vi "basic - Board Configuration.vi"() -> ()   [LabVIEW 2020]
uses:
  _controls/initialize_ExpertMode.ctl
  _controls/initialize_PortSpeed.ctl
  _controls/initialize_PortConfig.ctl
  AIM664LV.lvlib
panel:
  out "BSP Version Parameters":string[][](table)
  in  "ARINC 664 Resources":string[](tree)
  in  "Server Name":string="local"
  out "NuOfResources":u32
  out "new config":bool
  out "Board Control Out":T1 {"SharedMemFree" format="%x"; "GlobalMemFree" format="%x"; "ExpertMode" items=["FDX_EXPERT_MODE", "FDX_DISA_GHOST"]; "PortGoodLink" items=["FDX_NO_LINK", "FDX_GOOD_LINK"]; "PortSpeed" items=["FDX_100MBIT", "FDX_10MBIT", "FDX_AUTO_100MBIT", "FDX_AUTO_10MBIT", "FDX_AUTO_ERROR", "FDX_1000MBIT"]; "PortConfig" items=["FDX_SINGLE", "FDX_REDUNDANT"]}
  out "BSP Version Out":T2
  out "timed out":bool
  in  "PortConfig (single)":T3 {"Port1ConfigIn" items=["FDX_SINGLE", "FDX_REDUNDANT"]; "Port2ConfigIn" items=["FDX_SINGLE", "FDX_REDUNDANT"]; "Port3ConfigIn" items=["FDX_SINGLE", "FDX_REDUNDANT"]; "Port4ConfigIn" items=["FDX_SINGLE", "FDX_REDUNDANT"]}
  in  "PortSpeed (100Mbit)":T4 {"Port4SpeedIn" items=["FDX_100MBIT"=0, "FDX_10MBIT"=1, "FDX_AUTO_100MBIT"=2, "FDX_AUTO_10MBIT"=3, "FDX_1000MBIT"=5]; "Port3SpeedIn" items=["FDX_100MBIT"=0, "FDX_10MBIT"=1, "FDX_AUTO_100MBIT"=2, "FDX_AUTO_10MBIT"=3, "FDX_1000MBIT"=5]; "Port2SpeedIn" items=["FDX_100MBIT"=0, "FDX_10MBIT"=1, "FDX_AUTO_100MBIT"=2, "FDX_AUTO_10MBIT"=3, "FDX_1000MBIT"=5]; "Port1SpeedIn" items=["FDX_100MBIT"=0, "FDX_10MBIT"=1, "FDX_AUTO_100MBIT"=2, "FDX_AUTO_10MBIT"=3, "FDX_1000MBIT"=5]}
  in  "ExpertMode(ExpertMode)":T5 {"Expert1Mode" items=["FDX_EXPERT_MODE", "FDX_DISA_GHOST"]; "Expert2Mode" items=["FDX_EXPERT_MODE", "FDX_DISA_GHOST"]; "Expert3Mode" items=["FDX_EXPERT_MODE", "FDX_DISA_GHOST"]; "Expert4Mode" items=["FDX_EXPERT_MODE", "FDX_DISA_GHOST"]}
  out "error out":errorcluster
  in  "board index":i32
  # "ARINC 664 Board Control"
  # "Overview: Queries the boards available in a system and present some properties of those resources.\nRequirement: At least one AIM ARINC-664 board with installed AIM ARINC 664 BSP.\nRestrictions: None.\nInstruction:\n1. Select port to open based on port and board index values\n2. configure Pors Speed, PortConfig and ExpertMode fore each port\n3. Run the VI\n4. Check the BSP version out and Board Control Out indicator. new config led will turn on if a new configuration is applied, otherwise nothing will be changed"
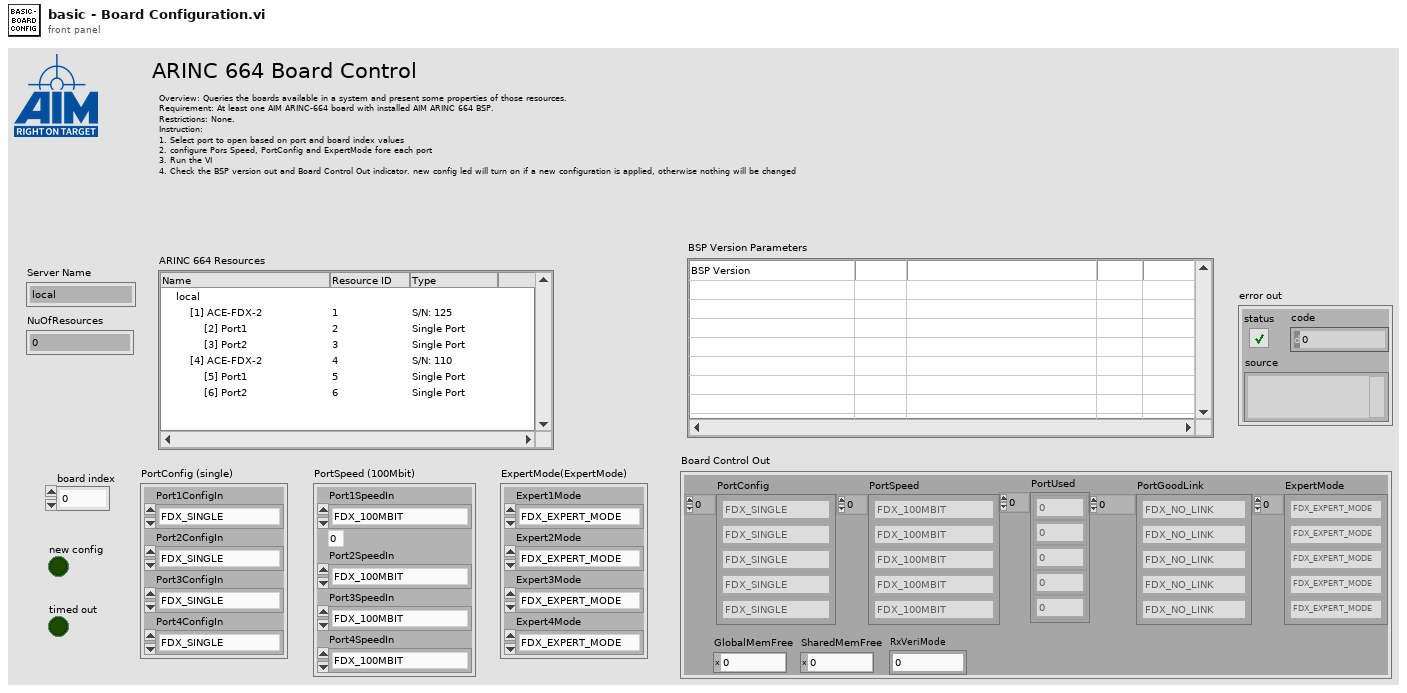
[diagram p1: front panel]
types:
  T1 = cluster{"PortConfig":u32[], "PortSpeed":u32[], "PortUsed":u32[], "PortGoodLink":u32[], "ExpertMode":u32[], "GlobalMemFree":u32, "SharedMemFree":u32, "RxVeriMode":u32}
  T2 = cluster{"SysDrvMajorVer":u32, "SysDrvMinorVer":u32, "SysDrvBuildNr":u32, "DllMajorVer":u32, "DllMinorVer":u32, "DllBuildNr":u32, "TargetMajorVer":u32, "TargetMinorVer":u32, "TargetBuildNr":u32, "FirmwareBiu1MajorVer":u32, "FirmwareBiu1MinorVer":u32, "FirmwareBiu1BuildNr":u32, "FirmwareBiu2MajorVer":u32, "FirmwareBiu2MinorVer":u32, "FirmwareBiu2BuildNr":u32, "MainLcaMajorVer":u32, "MainLcaMinorVer":u32, "MainLcaBuildNr":u32, "LcaBiu1MajorVer":u32, "LcaBiu1MinorVer":u32, "LcaBiu2MajorVer":u32, "LcaBiu2MinorVer":u32, "PciLcaMajorVer":u32, "PciLcaMinorVer":u32, "TcpMajorVer":u32, "TcpMinorVer":u32, "BootstrapMajorVer":u32, "BootstrapMinorVer":u32, "MonitorMajorVer":u32, "MonitorMinorVer":u32, "TargetOSMajor":u32, "TargetOSMinor":u32, "BspCompatibility":u32}
  T3 = typedef "AIM664LV.lvlib/initialize_PortConfig.ctl" = cluster{"Port1ConfigIn":u32, "Port2ConfigIn":u32, "Port3ConfigIn":u32, "Port4ConfigIn":u32}
  T4 = typedef "AIM664LV.lvlib/initialize_PortSpeed.ctl" = cluster{"Port1SpeedIn":u32, "Port2SpeedIn":u32, "Port3SpeedIn":u32, "Port4SpeedIn":u32}
  T5 = typedef "AIM664LV.lvlib/initialize_ExpertMode.ctl" = cluster{"Expert1Mode":u32, "Expert2Mode":u32, "Expert3Mode":u32, "Expert4Mode":u32}
  T6 = cluster{"BoardName":string, "BoardSerialNo":u32, "BoardNumOf\nEthernetPorts":u32, "BoardClients":u32, "BoardGlobal\nMemSize":u32, "BoardShared\nMemSize":u32, "BoardStructId":u32, "PortName":string, "PortMode":u32, "PortNo":u32, "PortBoard\nResourceID":u32, "PortStructId":u32}
  T7 = cluster{"Left Cell String":string, "Child Text":string[], "Child Tag":string, "Item Indent":i32, "Child Only?":bool, "Glyph Index":i32}
  T8 = cluster{"Left Cell String":string, "Child Text":string[], "Child Tag":string, "Item Indent":i32, "Child Only?":bool, "Glyph Index":i32}[]
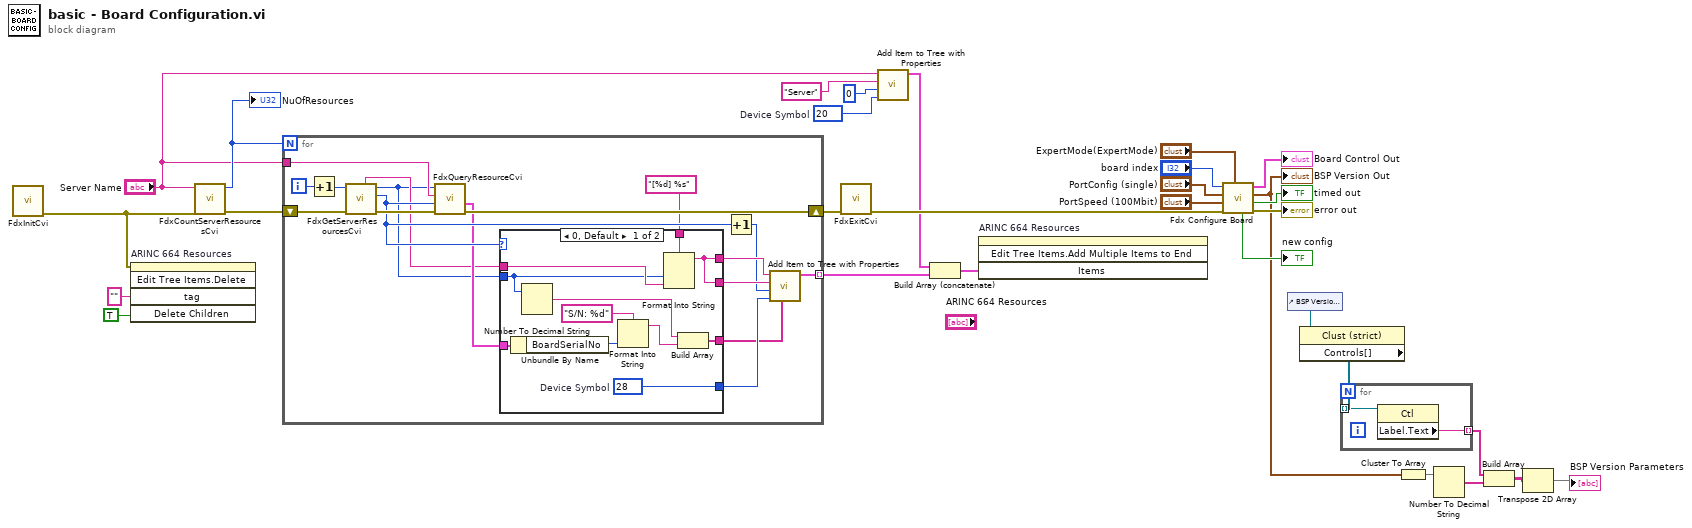
[diagram p0: block diagram]
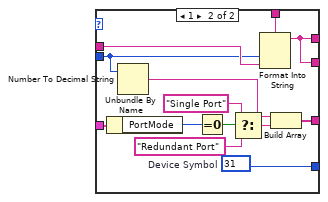
[diagram p2: hidden frame]
diagram:
  w17 = 20  # Device Symbol
  n1 = call "FdxInitCvi.vi"() -> ("error out"=w12:errorcluster)  [unwired: 10 in, 1 out]
  n2 = invoke on="ARINC 664 Resources" class="Tree (strict)" method="Edit Tree Items.Delete"(error in=w12, "tag"="" ("Tag"), "Delete Children"=TRUE ("Delete Children?")) -> ()  [unwired: 2 in, 5 out]
  n3 = call "FdxCountServerResourcesCvi.vi"("error in"=w12, "SrvName (local)"="Server Name") -> ("error out"=w21:errorcluster, "Number of Resources"=w20:u32)  [unwired: 8 in]
  "NuOfResources" <- w20
  n4 = for {
    N: w20 -> [_]
    shift-right: [w40] -> w9
    shift-left: w21 -> [w47]
    tunnel: [w44] -> w19 mode=indexing
    tunnel: "Server Name" -> [w39]
    i -> [w45]
    n5 = Increment(x=w45) -> (x+1=w42:i32)
    n6 = call "FdxGetServerResourcesCvi.vi"("error in"=w47, "ServerRElement"=w42) -> ("error out"=w41:errorcluster, "ResourceType"=w38:u32, "Resource ID"=w35:u32, "Resource Info"=w36:string)  [unwired: 4 in, 2 out]
    n7 = call "FdxQueryResourceCvi.vi"("error in"=w41, "ResourceType"=w38, "SrvName"=w39, "ResourceID"=w35) -> ("error out"=w40:errorcluster, "ResourceInfo"=w37:T6)  [unwired: 5 in, 1 out]
    n8 = case shown="0, Default" w38 {
      tunnel: [w58 w71] -> w46
      tunnel: [w50 w61] -> w43
      tunnel: w37 -> [w55 w68]
      tunnel: w36 -> [w57 w69]
      tunnel: w35 -> [w49 w59]
      tunnel: [w50 w61] -> w34
      tunnel: "[%d] %s" ("format string") -> [w56 w70]
      tunnel: [w54 w62] -> w32
      frame 0, Default {
        w58 = 28  # Device Symbol
        n9 = Unbundle By Name(w55) -> ("BoardSerialNo"=w53:u32)
        n10 = Number To Decimal String(number=w49) -> (decimal integer string=w48:string)  [unwired: 1 in]
        n11 = Format Into String(format string="S/N: %d", w53) -> (resulting string=w52:string)  [unwired: 2 in, 1 out]
        n12 = Format Into String(format string=w56, w49, w57) -> (resulting string=w50:string)  [unwired: 2 in, 1 out]
        n13 = Build Array(w48, w52) -> (w54:string[])
      }
      frame 1 {
        w71 = 31  # Device Symbol
        n14 = Unbundle By Name(w68) -> ("PortMode"=w67:u32)
        n15 = Number To Decimal String(number=w59) -> (decimal integer string=w60:string)  [unwired: 1 in]
        n16 = Equal To 0?(x=w67) -> (x = 0?=w66:bool)
        n17 = Select(t="Single Port" ("Child Tag"), s=w66, f="Redundant Port" ("Child Tag")) -> (s? t:f=w65:string)
        n18 = Format Into String(format string=w70, w59, w69) -> (resulting string=w61:string)  [unwired: 2 in, 1 out]
        n19 = Build Array(w60, w65) -> (w62:string[])
      }
    }
    n20 = Increment(x=w38) -> (x+1=w31:u32)
    n21 = call "Add Item to Tree with Properties.vi"("Child Text"=w32, "Glyph Index"=w46, "Item indent"=w31, "Child Tag"=w43, "Left Cell String"=w34) -> ("Item"=w44:T7)  [unwired: 6 in]
  }
  n22 = call "FdxExitCvi.vi"("error in"=w9) -> ("error out"=w22:errorcluster)  [unwired: 10 in]
  n23 = call "Add Item to Tree with Properties.vi"("Glyph Index"=w17, "Item indent"=0, "Child Tag"="Server", "Left Cell String"="Server Name") -> ("Item"=w18:T7)  [unwired: 7 in]
  n24 = Build Array (concatenate)(w18, w19) -> (w13:T8)
  n25 = invoke on="ARINC 664 Resources" class="Tree (strict)" method="Edit Tree Items.Add Multiple Items to End"("Items"=w13) -> ()  [unwired: 3 in, 4 out]
  n26 = call "Fdx Configure Board.vi"("ExpertMode(ExpertMode)"="ExpertMode(ExpertMode)", "error in (no error)"=w22, "PortSpeed (100Mbit)"="PortSpeed (100Mbit)", "PortConfig (single)"="PortConfig (single)", "board index"="board index") -> ("error out"=→"error out":errorcluster, "timed out"=→"timed out":bool, "BSP Version Out"=w1:T2, "Board Control Out"=→"Board Control Out":T1, "new config"=→"new config":bool)  [unwired: 2 in]
  "BSP Version Out" <- w1
  n27 = control-ref of="BSP Version Out"() -> (w2:refnum<vi>)
  n28 = property on="Property Node" class="Clust (strict)"(reference=w2) -> ("Controls[]"=w4:refnum<vi>[])  [unwired: 1 in, 2 out]
  n29 = for {
    tunnel: w4 -> [w73] mode=indexing
    tunnel: [w72] -> w3 mode=indexing
    n30 = property class="Ctl"(reference=w73) -> ("Label.Text"=w72:string)  [unwired: 1 in, 2 out]
  }
  n31 = Cluster To Array(cluster=w1) -> (array=w8:u32[])
  n32 = Number To Decimal String(number=w8) -> (decimal integer string=w7:string[])  [unwired: 1 in]
  n33 = Build Array(w3, w7) -> (w6:string[][])
  n34 = Transpose 2D Array(2D array=w6) -> (transposed array=→"BSP Version Parameters":string[][])
